vi "FPGA实物信号仿真 - 副本.vi"() -> ()   [LabVIEW 2012]
uses:
  P3060NEW/_SubVI/dll/Release/P3060.dll
panel:
  out "时域/频域切换":bool
  in  "设置按钮":bool
  out "数据采集次数":i32
  in  "板卡单次传输点数":u32=8192
  out "error out":errorcluster caption="错误输出"
  in  "槽位号":i16=5
  in  "取消按钮":bool
  in  "FPGA-Bit文件路径":path
  in  "加载程序":bool caption="确定按钮"
  out "波形图":i32[](graph)
  in  "read":bool caption="显示采集卡数据"
  in  "板卡LED控制":bool
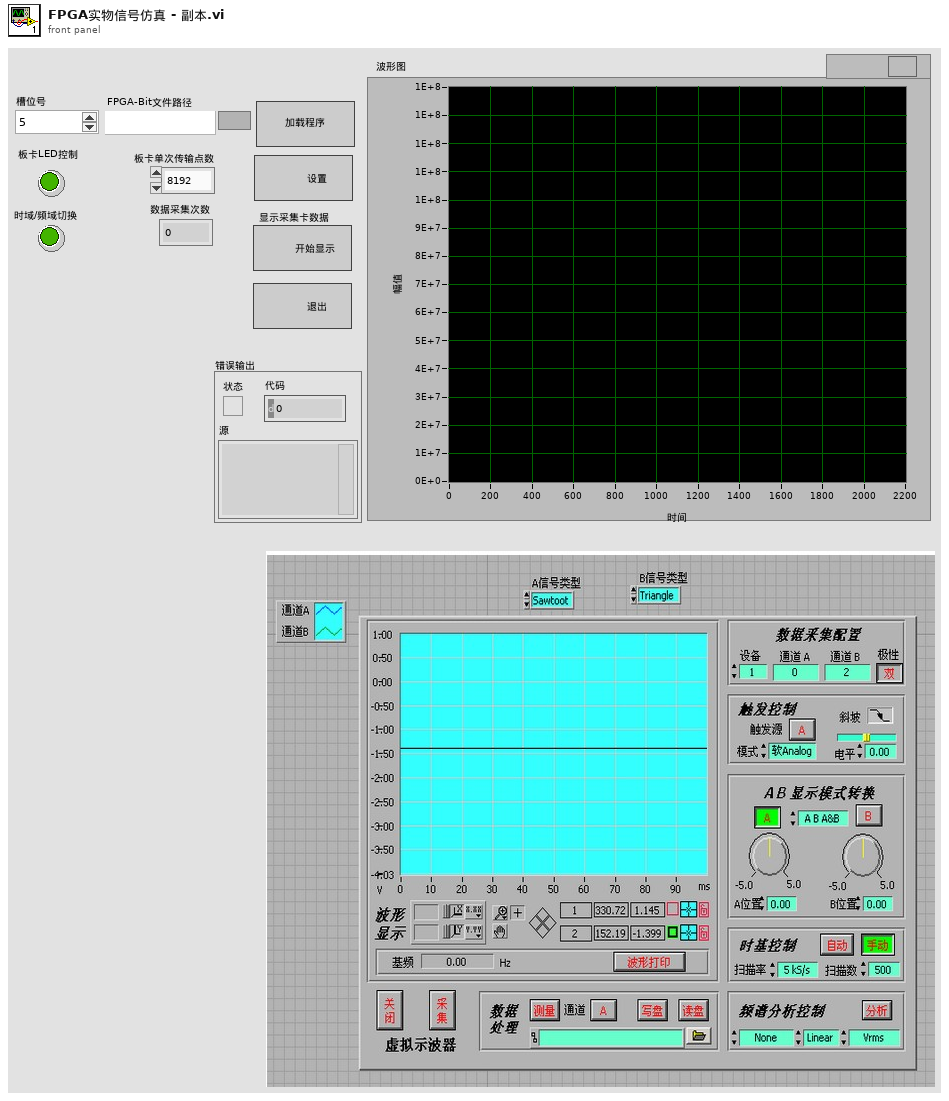
[diagram p1: front panel]
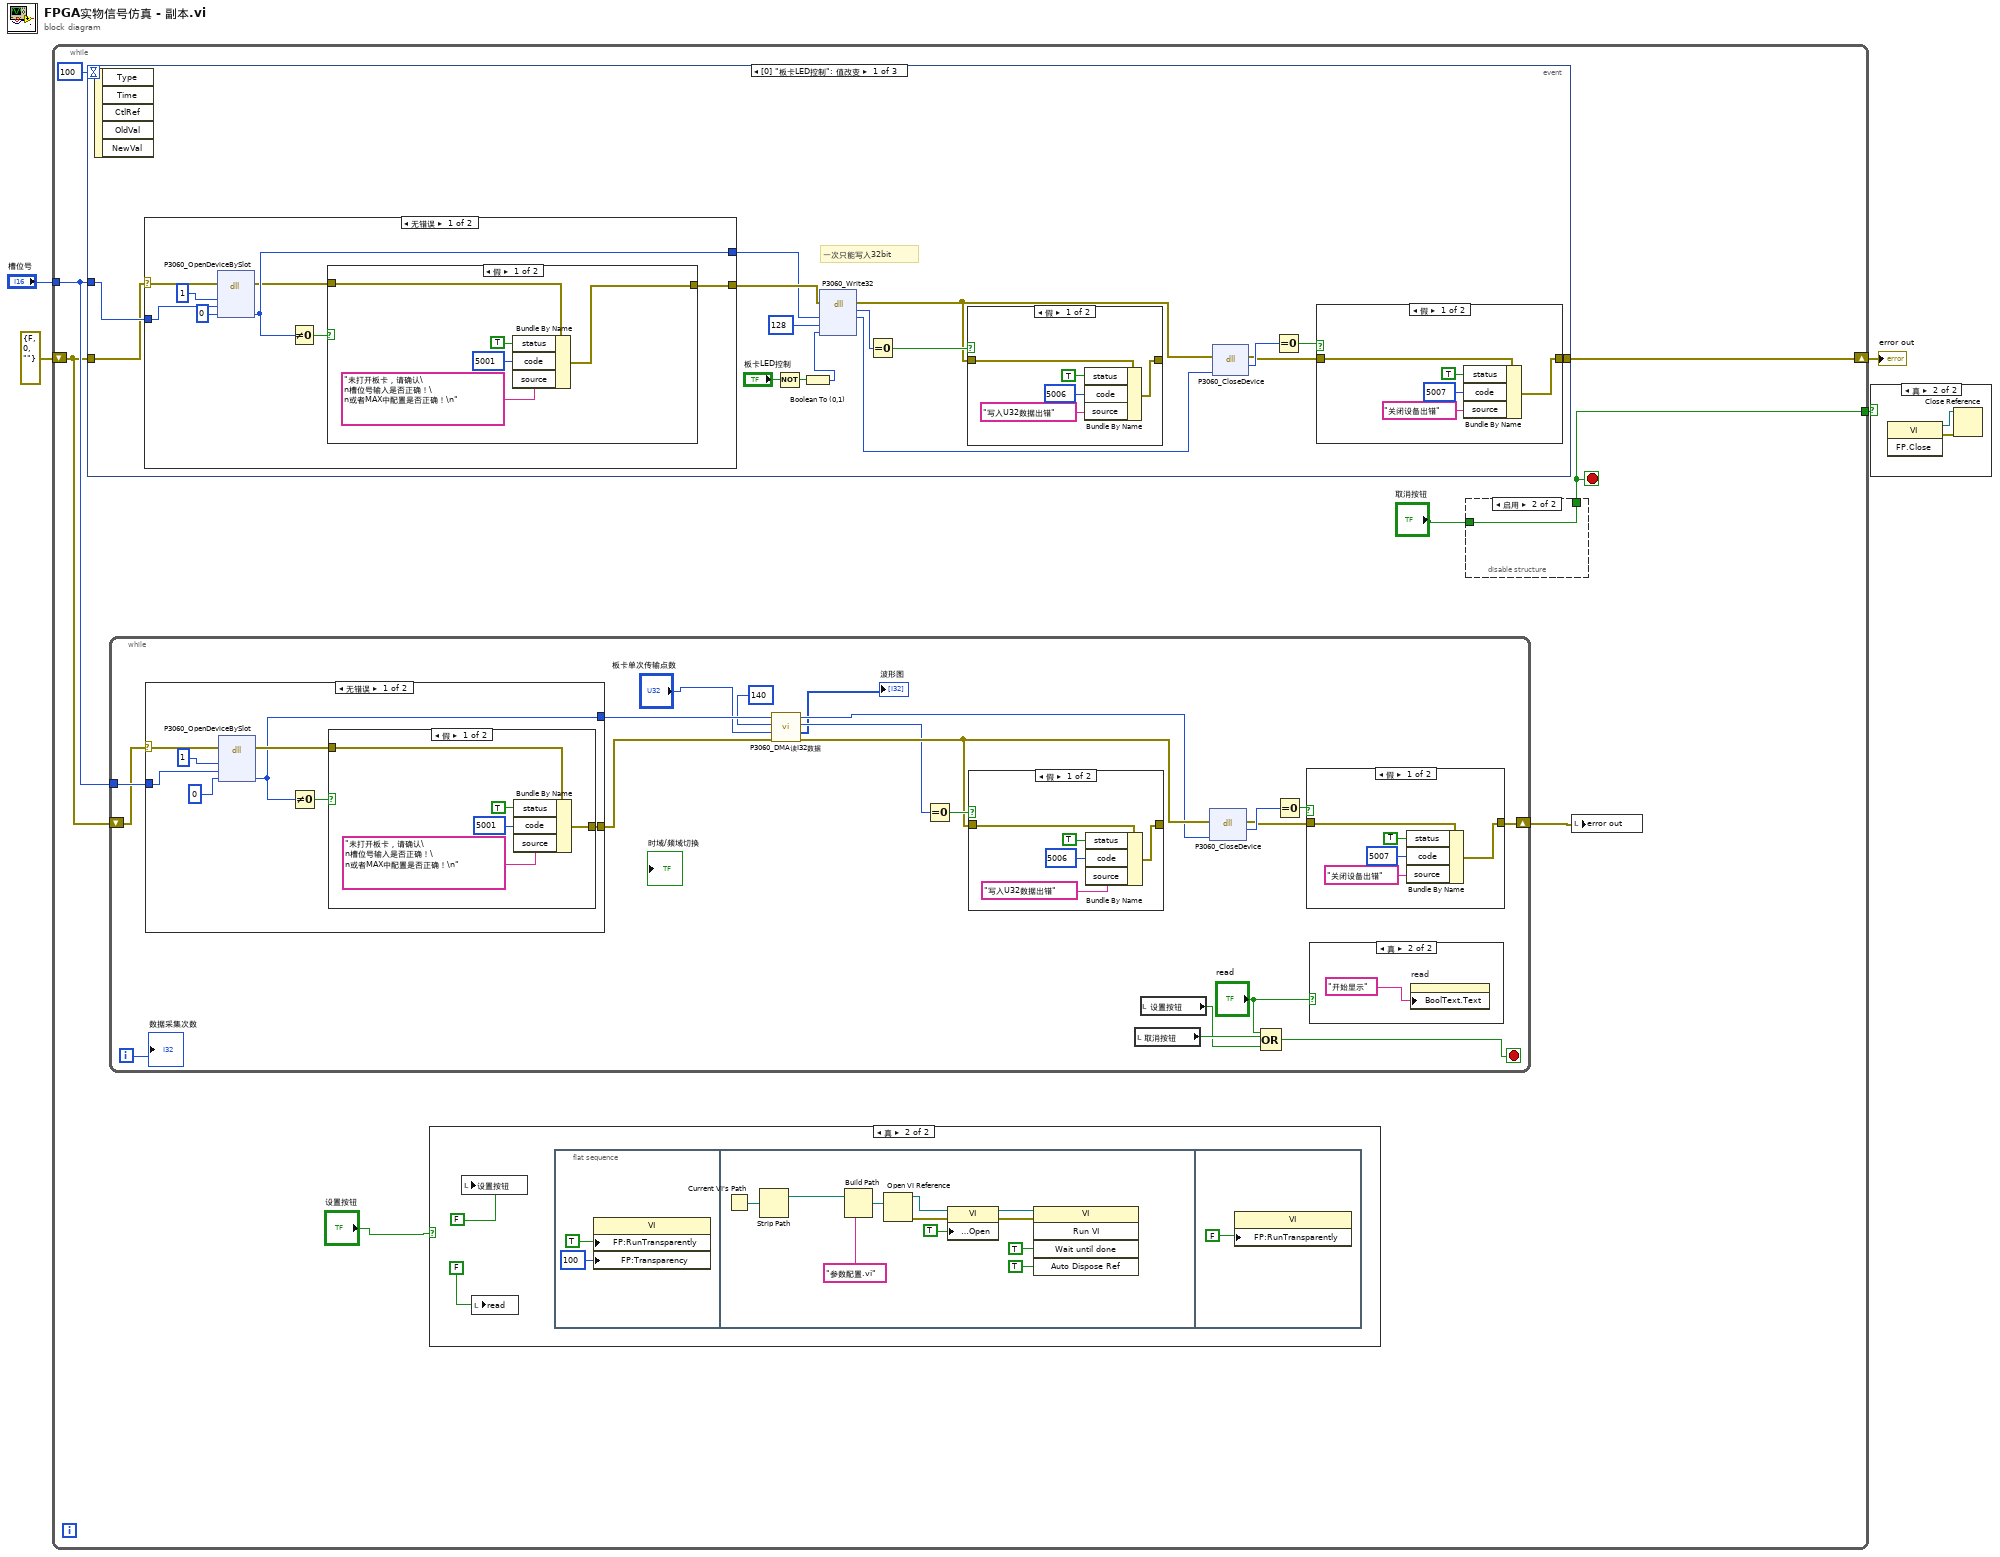
[diagram p0: block diagram]
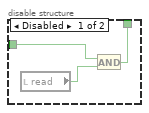
[diagram p3: hidden frame]
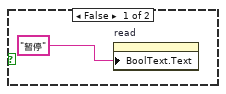
[diagram p4: hidden frame]
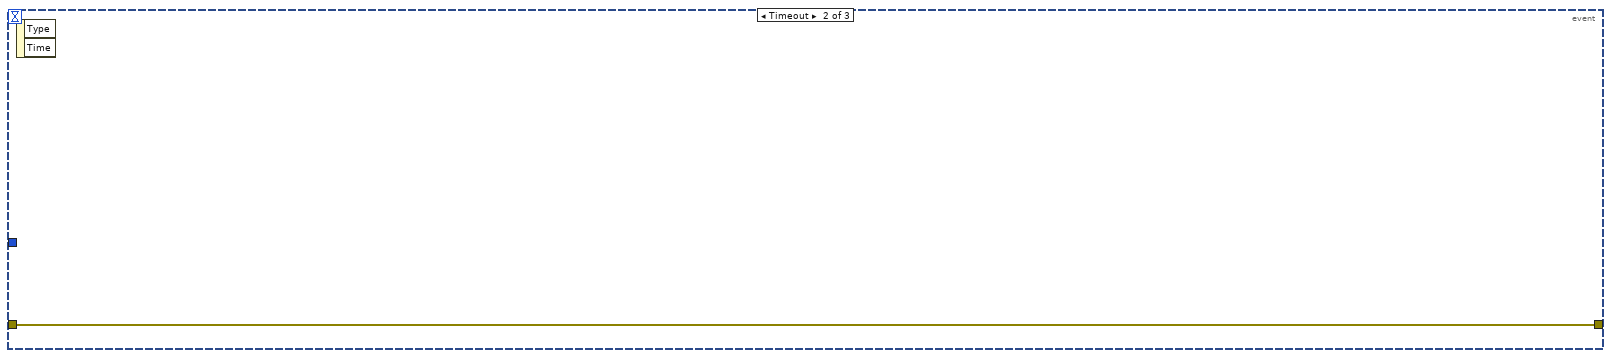
[diagram p13: hidden frame]
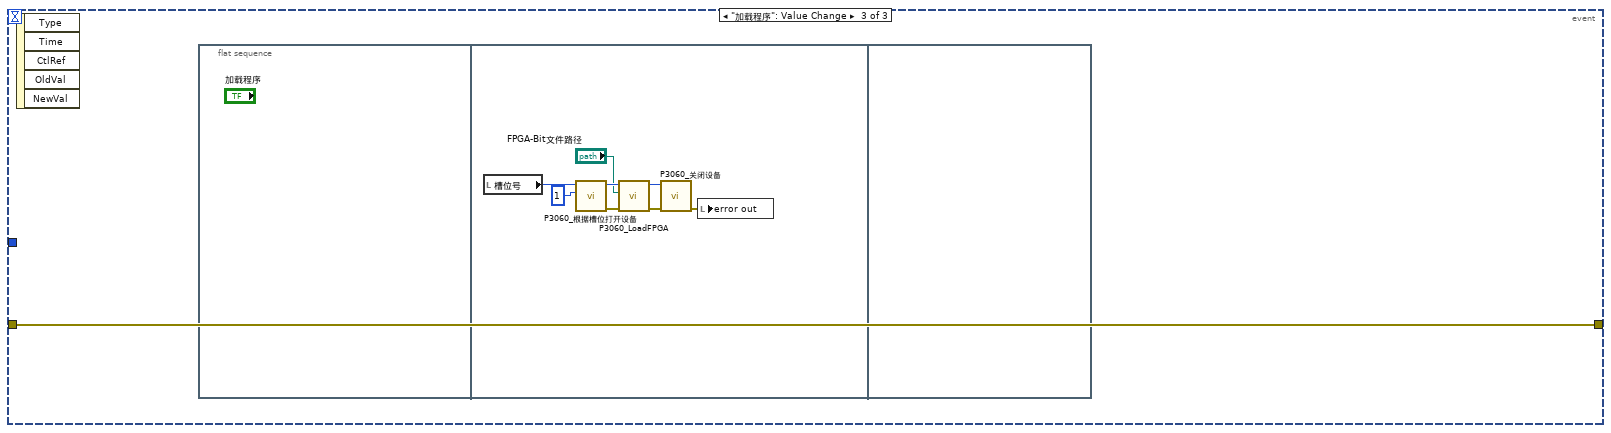
[diagram p14: hidden frame]
diagram:
  n1 = while {
    tunnel: "槽位号" -> [w10]
    shift-right: [w12] -> w2
    shift-left: errorcluster {"status"=FALSE, "code"=0, "source"=""} ("error IO") -> [w6]
    tunnel: [w8] -> w1
    stop <- w8 stop-if-true
    n2 = event shown="[0] \"板卡LED控制\": 值改变" {
      selector: _ -> [_ _ _]
      dyn-events: _ -> [_ _ _]
      timeout: 100 -> [_ _ _]
      tunnel: w10 -> [w87 _ _]
      tunnel: [w85 w125 w126] -> w12
      tunnel: w6 -> [w86 w125 w126]
      event "板卡LED控制": Value Change {
        # "一次只能写入32bit"
        n3 = event-data() -> ()  [unwired: 1 in, 5 out]
        n4 = case shown="无错误" w86 {
          selector: w86 -> [w117 w124]
          tunnel: [w114 w124] -> w92
          tunnel: w87 -> [w116 _]
          tunnel: [w113 _] -> w90
          frame No Error {
            n5 = dll-call lib="C:/PLC_simulation/2014.2.25PLC_NEW/PLC_NEW/P3060NEW/_SubVI/dll/Release/P3060.dll" fn="P3060_OpenDeviceBySlot"(error in=w117, "Classis"=i16 1, "槽位号"=w116, "设备句柄"=0) -> (error out=w110:errorcluster, "设备句柄"=w113:i32)  [unwired: 5 in, 1 out]
            n6 = Not Equal To 0?(x=w113) -> (x != 0?=w115:bool)
            n7 = case shown="假" w115 {
              tunnel: w110 -> [w122 w123]
              tunnel: [w118 w123] -> w114
              frame False {
                n8 = Bundle By Name(cluster=w122, "status"=TRUE, "code"=5001, "source"="未打开板卡，请确认\n槽位号输入是否正确！\n或者MAX中配置是否正确！\n") -> (w118:errorcluster)
              }
              frame True {
              }
            }
          }
          frame Error {
          }
        }
        n9 = Not(x="板卡LED控制") -> (.not. x?=w83:bool)
        n10 = Boolean To (0,1)(Boolean=w83) -> (0, 1=w84:i16)
        n11 = dll-call lib="C:/PLC_simulation/2014.2.25PLC_NEW/PLC_NEW/P3060NEW/_SubVI/dll/Release/P3060.dll" fn="P3060_Write32"(error in=w92, "hDev"=w90, "Offset"=u32 128, "data"=w84) -> (error out=w91:errorcluster, "return"=w94:i32, "hDev"=w89:i32)  [unwired: 4 in, 1 out]
        n12 = Equal To 0?(x=w94) -> (x = 0?=w93:bool)
        n13 = case shown="假" w93 {
          tunnel: [w101 w103] -> _
          tunnel: w91 -> [w102 w103]
          frame False {
            n14 = Bundle By Name(cluster=w102, "status"=TRUE, "code"=5006, "source"="写入U32数据出错") -> (w101:errorcluster)
          }
          frame True {
          }
        }
        n15 = dll-call lib="C:/PLC_simulation/2014.2.25PLC_NEW/PLC_NEW/P3060NEW/_SubVI/dll/Release/P3060.dll" fn="P3060_CloseDevice"(error in=w91, "hDev"=w89) -> (error out=w95:errorcluster, "hDevOut"=w97:i32)  [unwired: 3 in, 1 out]
        n16 = Equal To 0?(x=w97) -> (x = 0?=w96:bool)
        n17 = case shown="假" w96 {
          tunnel: [w107 w109] -> w85
          tunnel: w95 -> [w108 w109]
          frame False {
            n18 = Bundle By Name(cluster=w108, "status"=TRUE, "code"=5007, "source"="关闭设备出错") -> (w107:errorcluster)
          }
          frame True {
          }
        }
      }
      event Timeout {
        n19 = event-data() -> ()  [unwired: 1 in, 2 out]
      }
      event "加载程序": Value Change {
        n20 = event-data() -> ()  [unwired: 1 in, 5 out]
        n21 = flat-sequence {
          frame #0 {
          }
          frame #1 {
            n22 = local read "槽位号"() -> (w134:i16)
            n23 = call "P3060_根据槽位打开设备.vi"("机箱号"=i16 1, "槽位号"=w134) -> ("error out"=w130:errorcluster, "句柄输出"=w128:i32)  [unwired: 8 in]
            n24 = call "P3060_LoadFPGA.vi"("错误输入"=w130, "Bit文件路径"="FPGA-Bit文件路径", "句柄输入"=w128) -> ("错误输出"=w132:errorcluster, "句柄输出"=w131:i32)  [unwired: 6 in, 1 out]
            n25 = call "P3060_关闭设备.vi"("error in (no error)"=w132, "句柄输入"=w131) -> ("error out"=w133:errorcluster)  [unwired: 9 in]
            n26 = local write "error out"(w133) -> ()
          }
          frame #2 {
          }
        }
      }
    }
    n27 = while {
      tunnel: w10 -> [w42]
      shift-right: [w38] -> w7
      shift-left: w6 -> [w37]
      i -> [w39]
      stop <- w34 stop-if-true
      n28 = case shown="无错误" w37 {
        selector: w37 -> [w74 w81]
        tunnel: [w70 w81] -> w47
        tunnel: w42 -> [w73 _]
        tunnel: [w67 _] -> w48
        frame No Error {
          n29 = dll-call lib="C:/PLC_simulation/2014.2.25PLC_NEW/PLC_NEW/P3060NEW/_SubVI/dll/Release/P3060.dll" fn="P3060_OpenDeviceBySlot"(error in=w74, "Classis"=i16 1, "槽位号"=w73, "设备句柄"=0) -> (error out=w71:errorcluster, "设备句柄"=w67:i32)  [unwired: 5 in, 1 out]
          n30 = Not Equal To 0?(x=w67) -> (x != 0?=w72:bool)
          n31 = case shown="假" w72 {
            tunnel: w71 -> [w79 w80]
            tunnel: [w75 w80] -> w70
            frame False {
              n32 = Bundle By Name(cluster=w79, "status"=TRUE, "code"=5001, "source"="未打开板卡，请确认\n槽位号输入是否正确！\n或者MAX中配置是否正确！\n") -> (w75:errorcluster)
            }
            frame True {
            }
          }
        }
        frame Error {
        }
      }
      n33 = call "P3060_DMA读I32数据.vi"("错误输入"=w47, "数据长度"="板卡单次传输点数", "偏移地址"=u32 140, "句柄输入"=w48) -> ("错误输出"=w46:errorcluster, "读I32数据"=→"波形图":i32[], "返回值"=w45:i32, "句柄输出"=w44:i32)  [unwired: 4 in]
      n34 = Equal To 0?(x=w45) -> (x = 0?=w49:bool)
      n35 = case shown="假" w49 {
        tunnel: [w58 w60] -> _
        tunnel: w46 -> [w59 w60]
        frame False {
          n36 = Bundle By Name(cluster=w59, "status"=TRUE, "code"=5006, "source"="写入U32数据出错") -> (w58:errorcluster)
        }
        frame True {
        }
      }
      n37 = local read "取消按钮"() -> (w35:bool)
      n38 = local read "设置按钮"() -> (w33:bool)
      n39 = dll-call lib="C:/PLC_simulation/2014.2.25PLC_NEW/PLC_NEW/P3060NEW/_SubVI/dll/Release/P3060.dll" fn="P3060_CloseDevice"(error in=w46, "hDev"=w44) -> (error out=w50:errorcluster, "hDevOut"=w52:i32)  [unwired: 3 in, 1 out]
      n40 = Compound Arithmetic op=OR("read", w35, w33) -> (w34:bool)
      n41 = Equal To 0?(x=w52) -> (x = 0?=w51:bool)
      n42 = case shown="假" w51 {
        tunnel: [w64 w66] -> w38
        tunnel: w50 -> [w65 w66]
        frame False {
          n43 = Bundle By Name(cluster=w65, "status"=TRUE, "code"=5007, "source"="关闭设备出错") -> (w64:errorcluster)
        }
        frame True {
        }
      }
      n44 = case shown="真" "read" {
        frame False {
          n45 = property on="read" class="Bool (严格)"("BoolText.Text"="暂停") -> ()  [unwired: 2 in, 2 out]
        }
        frame True {
          n46 = property on="read" class="Bool (严格)"("BoolText.Text"="开始显示") -> ()  [unwired: 2 in, 2 out]
        }
      }
      "数据采集次数" <- w39
    }
    n47 = case shown="真" "设置按钮" {
      frame False {
      }
      frame True {
        n48 = local write "设置按钮"(FALSE ("布尔")) -> ()
        n49 = local write "read"(FALSE) -> ()
        n50 = flat-sequence {
          frame #0 {
            n51 = property class="VI"("FP:RunTransparently"=TRUE ("前面板窗口:以透明方式运行VI"), "FP:Transparency"=u8 100 ("前面板窗口:透明度")) -> ()  [unwired: 2 in, 2 out]
          }
          frame #1 {
            n52 = Current VI's Path() -> (path=w17:path)
            n53 = Strip Path(path=w17) -> (stripped path=w27:path)  [unwired: 1 out]
            n54 = Build Path(base path=w27, name or relative path="参数配置.vi" ("名称或相对路径")) -> (appended path=w26:path)
            n55 = Open VI Reference(vi path=w26) -> (vi reference=w25:refnum<vi>, error out=w24:errorcluster)  [unwired: 5 in]
            n56 = property class="VI"(reference=w25, error in=w24, "Front Panel.Open"=TRUE ("前面板窗口:打开")) -> (reference out=w22:refnum<vi>, error out=w21:errorcluster)
            n57 = invoke class="VI" method="Run VI"(reference=w22, error in=w21, "Wait until done"=TRUE ("结束前等待"), "Auto Dispose Ref"=TRUE ("自动销毁引用")) -> ()  [unwired: 1 in, 5 out]
          }
          frame #2 {
            n58 = property class="VI"("FP:RunTransparently"=FALSE ("前面板窗口:以透明方式运行VI")) -> ()  [unwired: 2 in, 2 out]
          }
        }
      }
    }
    n59 = disable-structure shown="启用" {
      disable-tunnel: "取消按钮" -> [w30 w32]
      disable-tunnel: [w29 w32] -> w8
      frame Disabled {
        n60 = local read "read"() -> (w31:bool)
        n61 = And(x=w30, y=w31) -> (x .and. y?=w29:bool)
      }
      frame Enabled {
      }
    }
    n62 = local write "error out"(w7) -> ()
  }
  "error out" <- w2
  n63 = case shown="真" w1 {
    frame False {
    }
    frame True {
      n64 = invoke class="VI" method="FP.Close"() -> (reference out=w135:refnum<vi>, error out=w136:errorcluster)  [unwired: 3 in, 1 out]
      n65 = Close Reference(reference=w135, error in (no error)=w136) -> ()  [unwired: 1 out]
    }
  }
